vi "Read Max Qorf DVR.vi"(8 "error in (no error)":errorcluster, 11 "Get Max Orifice Flow in":refnum<class "Get Max Orifice Flow.lvclass">) -> (0 "error out":errorcluster, 2 "Max Qorf DVR":refnum<data-value>, 3 "Get Max Orifice Flow out":refnum<class "Get Max Orifice Flow.lvclass">)   [LabVIEW 2015, in "Get Max Orifice Flow.lvclass"]
uses:
  Get Max Orifice Flow.lvclass
  Get Max Orifice Flow.lvclass/Get Max Orifice Flow.ctl
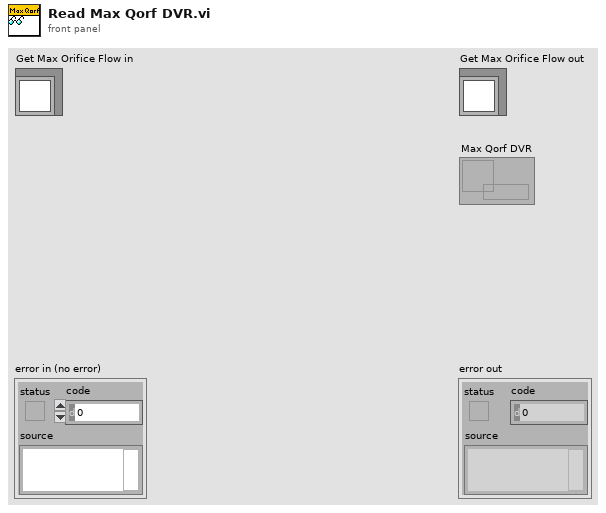
[diagram p1: front panel]
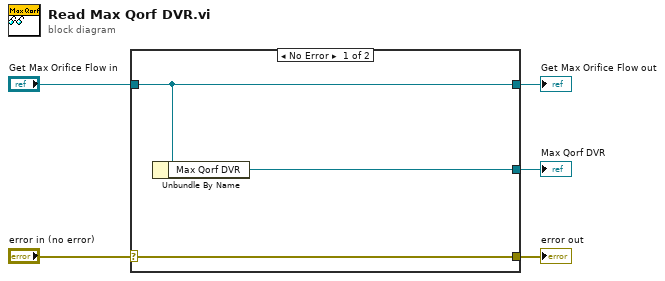
[diagram p0: block diagram]
diagram:
  n1 = case shown="No Error" "error in (no error)" {
    selector: "error in (no error)" -> [w8 w9]
    tunnel: [w8 w9] -> w4
    tunnel: [w7 w10] -> w2
    tunnel: "Get Max Orifice Flow in" -> [w7 w10]
    tunnel: [w6 _] -> w1
    frame No Error {
      n2 = Unbundle By Name(w7) -> ("Max Qorf DVR"=w6:refnum<data-value>)
    }
    frame Error {
    }
  }
  "error out" <- w4
  "Get Max Orifice Flow out" <- w2
  "Max Qorf DVR" <- w1
